vi "DFD IIR Notch Peak Design.vi"   [LabVIEW 2017, in "NI_DigFilterLicensed.lvlib"]
doc: "Designs a notch or peak filter in which the notch or peak is located at the center frequency. You must manually select the polymorphic instance you want to use."
uses:
  <vilib>/addons/Digital Filter Design/NI_DigFilterLicensed.lvlib
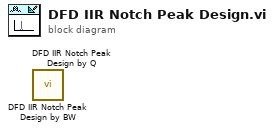
[diagram p0: block diagram]
diagram:
  n1 = call <vilib>:"DFD IIR Notch Peak Design by BW.vi"() -> ()  [unwired: 10 in, 2 out]
  n2 = call <vilib>:"DFD IIR Notch Peak Design by Q.vi"() -> ()  [unwired: 10 in, 2 out]
